vi "WillHeadingHitSegment.vi"(7 "Safety offset around edges (m)":dbl=5.0, 8 "Heading (deg)":dbl, 9 "Segment Point 2":T1 {"North" format="%#_10f"; "East" format="%#_8f"}, 10 "Segment Point 1":T1 {"North" format="%#_10f"; "East" format="%#_8f"}, 11 "Boat Point":T1 {"North" format="%#_10f"; "East" format="%#_8f"}) -> (3 "Will collide":bool)   [LabVIEW 2013, in "Obstacle.lvclass"]
doc: "This VI takes (boat position and heading), (two points for a line segment), and a safety offset. It then looks to see whether the given boat and heading will intersect the obstacle segments. This efectively expands the segment by the safety offset on each side, then checking whether the heading is within the two outer points.\n\nEric Schneider, August 2014"
uses:
  Obstacle.lvclass
  Data/TypeDefs/UTM Location.ctl
  Utilities/Math/Angles/Angle/Angle.lvclass
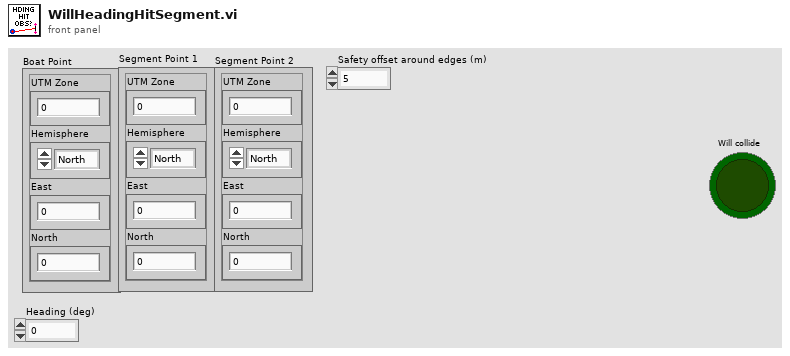
[diagram p1: front panel]
types:
  T1 = typedef "UTM Location.ctl" = cluster{"UTM Zone":dbl, "Hemisphere":enum16{"North", "South"}, "East":dbl, "North":dbl}
  T2 = cluster{"UTM Zone":dbl, "Hemisphere":u16, "East":dbl, "North":dbl}
  T3 = cluster{"UTM Zone":dbl, "Hemisphere":dbl, "East":dbl, "North":dbl}
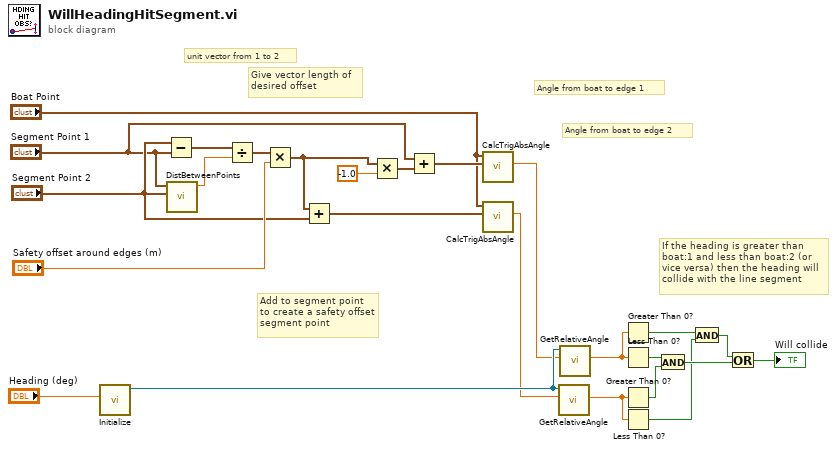
[diagram p0: block diagram]
diagram:
  # "If the heading is greater than boat:1 and less than boat:2 (or vice versa) then the heading will collide with the line segment"
  # "Angle from boat to edge 2"
  # "Angle from boat to edge 1"
  # "Add to segment point to create a safety offset segment point"
  # "Give vector length of desired offset"
  # "unit vector from 1 to 2"
  n1 = call "Initialize.vi"("Input Angle (Deg.)"="Heading (deg)") -> ("Angle out"=w15:refnum<class "Angle.lvclass">)  [unwired: 9 in, 1 out]
  n2 = Subtract(x="Segment Point 2", y="Segment Point 1") -> (x-y=w25:T2)
  n3 = call "DistBetweenPoints.vi"("UTM Location 2"="Segment Point 2", "UTM Location 1"="Segment Point 1") -> ("Distance from 1 to 2"=w24:dbl)  [unwired: 9 in]
  n4 = Divide(x=w25, y=w24) -> (x/y=w23:T3)
  n5 = Multiply(x=w23, y="Safety offset around edges (m)") -> (x*y=w19:T3)
  n6 = Add(x=w19, y="Segment Point 2") -> (x+y=w13:T3)
  n7 = Multiply(x=w19, y=-1.0) -> (x*y=w18:T3)
  n8 = Add(x="Segment Point 1", y=w18) -> (x+y=w14:T3)
  n9 = call "CalcTrigAbsAngle.vi"("Point 2"=w14, "Point 1"="Boat Point") -> ("Angle between points (deg)"=w11:dbl)  [unwired: 8 in, 1 out]
  n10 = call "CalcTrigAbsAngle.vi"("Point 2"=w13, "Point 1"="Boat Point") -> ("Angle between points (deg)"=w10:dbl)  [unwired: 8 in, 1 out]
  n11 = call "GetRelativeAngle.vi"("Boat Heading (Deg.)"=w10, "Angle in"=w15) -> ("Relative Angle"=w6:dbl)  [unwired: 7 in, 2 out]
  n12 = call "GetRelativeAngle.vi"("Boat Heading (Deg.)"=w11, "Angle in"=w15) -> ("Relative Angle"=w5:dbl)  [unwired: 7 in, 2 out]
  n13 = Greater Than 0?(x=w5) -> (x > 0?=w2:bool)
  n14 = Less Than 0?(x=w5) -> (x < 0?=w9:bool)
  n15 = Greater Than 0?(x=w6) -> (x > 0?=w8:bool)
  n16 = Less Than 0?(x=w6) -> (x < 0?=w3:bool)
  n17 = And(x=w9, y=w8) -> (x .and. y?=w7:bool)
  n18 = And(x=w2, y=w3) -> (x .and. y?=w4:bool)
  n19 = Or(x=w4, y=w7) -> (x .or. y?=→"Will collide":bool)
